vi "Uninitialize.vi"(8 "error in (no error)":errorcluster) -> (0 "error out":errorcluster)   [LabVIEW 2020, in "CodeSignAPI.lvlib"]
doc: "nicsgnUninit(void);"
uses:
  <vilib>/AppBuilder/CodeSignAPI/CodeSignAPI.lvlib
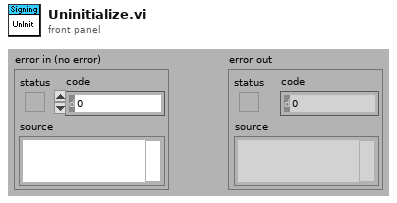
[diagram p1: front panel]
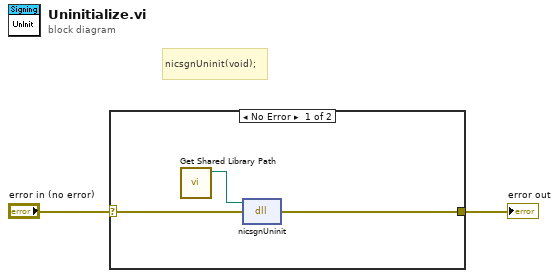
[diagram p0: block diagram]
diagram:
  # "nicsgnUninit(void);"
  n1 = case shown="No Error" "error in (no error)" {
    selector: "error in (no error)" -> [w4 w6]
    tunnel: [w5 w6] -> w2
    frame No Error {
      n2 = call <vilib>:"Get Shared Library Path.vi"() -> ("shared library path"=w3:path)  [unwired: 1 in, 10 out]
      n3 = dll-call lib="?" fn="nicsgnUninit"(path in=w3, error in=w4) -> (error out=w5:errorcluster)  [unwired: 1 in, 2 out]
    }
    frame Error {
    }
  }
  "error out" <- w2
